vi "Three Motor Mover.vi"() -> ()   [LabVIEW 2019]
panel:
  in  "Low 1":dbl=-100.0 format="%.1f"
  in  "High 1":dbl=100.0 format="%.1f"
  in  "Low 2":dbl=-100.0 format="%.1f"
  in  "High 2":dbl=100.0 format="%.1f"
  in  "Low 3":dbl=-100.0 format="%.1f"
  in  "High 3":dbl=100.0 format="%.1f"
  in  "Zero 3":bool
  in  "Zero 2":bool
  in  "Zero 1":bool
  out "Position 3":dbl format="%.4f"
  in  "Backward Big 3":bool
  in  "Forward Big 3":bool
  in  "Backward Small 3":bool
  in  "Forward Small 3":bool
  in  "Motor 3":refnum<visa-resource-name>="ASRL6::INSTR"
  in  "Large Step Size 3":dbl=10.0 format="%.1f"
  in  "Small Step Size 3":dbl=1.0 format="%_2f"
  out "Position 2":dbl format="%.4f"
  in  "Backward Big 2":bool
  in  "Forward Big 2":bool
  in  "Backward Small 2":bool
  in  "Forward Small 2":bool
  in  "Motor 2":refnum<visa-resource-name>="ASRL5::INSTR"
  in  "Large Step Size 2":dbl=10.0 format="%.1f"
  in  "Small Step Size 2":dbl=1.0 format="%_2f"
  out "Position 1":dbl format="%.4f"
  in  "stop":bool
  in  "Backward Big 1":bool
  in  "Forward Big 1":bool
  in  "Backward Small 1":bool
  in  "Forward Small 1":bool
  in  "Motor 1":refnum<visa-resource-name>="ASRL4::INSTR"
  in  "Large Step Size 1":dbl=10.0 format="%.1f"
  in  "Small Step Size 1":dbl=1.0 format="%_2f"
  # "Limits"
  # "Limits"
  # "Limits"
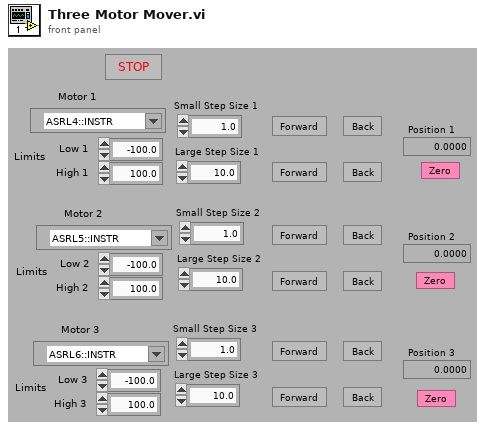
[diagram p1: front panel]
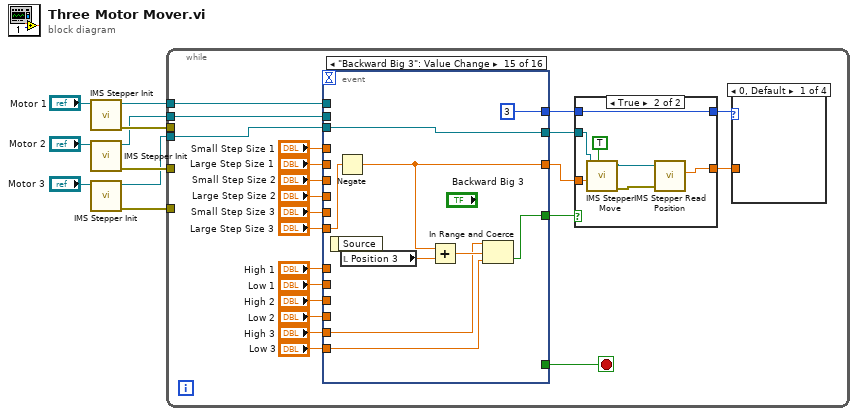
[diagram p0: block diagram]
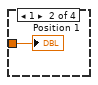
[diagram p2: hidden frame]
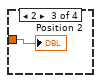
[diagram p3: hidden frame]
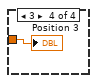
[diagram p4: hidden frame]
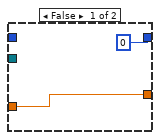
[diagram p5: hidden frame]
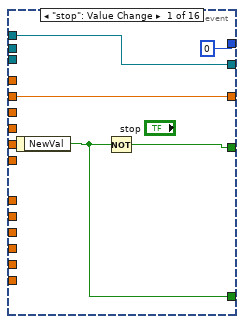
[diagram p6: hidden frame]
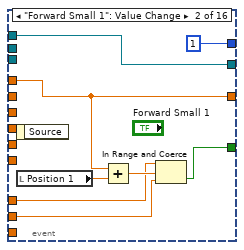
[diagram p7: hidden frame]
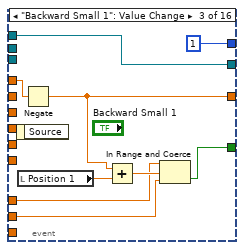
[diagram p8: hidden frame]
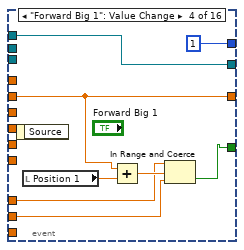
[diagram p9: hidden frame]
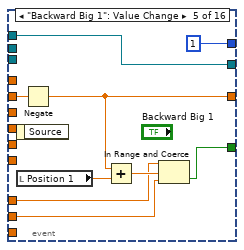
[diagram p10: hidden frame]
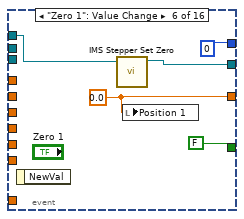
[diagram p11: hidden frame]
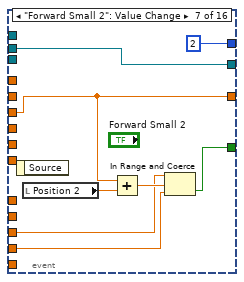
[diagram p12: hidden frame]
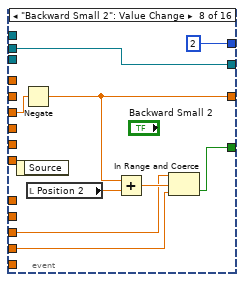
[diagram p13: hidden frame]
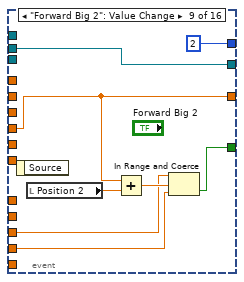
[diagram p14: hidden frame]
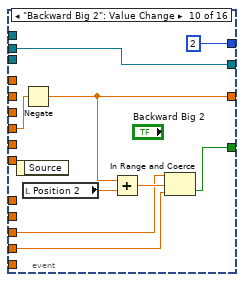
[diagram p15: hidden frame]
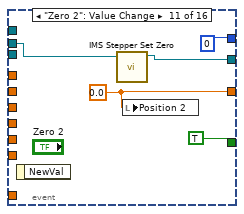
[diagram p16: hidden frame]
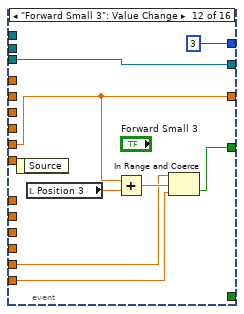
[diagram p17: hidden frame]
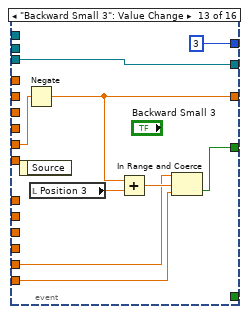
[diagram p18: hidden frame]
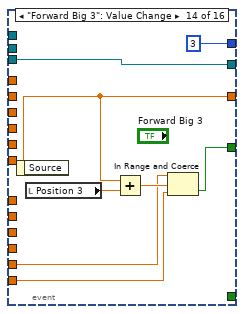
[diagram p19: hidden frame]
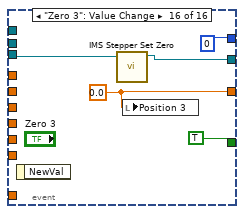
[diagram p20: hidden frame]
diagram:
  n1 = call "IMS Stepper Init.vi"("Instrument Address"="Motor 1") -> ("error out"=w9:errorcluster, "dup VISA Resource Name"=w5:refnum<visa-resource-name>)  [unwired: 4 in, 1 out]
  n2 = call "IMS Stepper Init.vi"("Instrument Address"="Motor 2") -> ("error out"=w7:errorcluster, "dup VISA Resource Name"=w3:refnum<visa-resource-name>)  [unwired: 4 in, 1 out]
  n3 = call "IMS Stepper Init.vi"("Instrument Address"="Motor 3") -> ("error out"=w8:errorcluster, "dup VISA Resource Name"=w1:refnum<visa-resource-name>)  [unwired: 4 in, 1 out]
  n4 = while {
    tunnel: w5 -> [w24]
    tunnel: w9 -> [_]
    tunnel: w8 -> [_]
    tunnel: w7 -> [_]
    tunnel: w3 -> [w22]
    tunnel: w1 -> [w21]
    stop <- w16 stop-if-true
    n5 = event shown="[14] \"Backward Big 3\": Value Change" {
      selector: _ -> [_ _ _ _ _ _ _ _ _ _ _ _ _ _ _ _]
      dyn-events: _ -> [_ _ _ _ _ _ _ _ _ _ _ _ _ _ _ _]
      timeout: _ -> [_ _ _ _ _ _ _ _ _ _ _ _ _ _ _ _]
      tunnel: w24 -> [w47 w56 w65 w73 w81 w84 _ _ _ _ _ _ _ _ _ _]
      tunnel: "Small Step Size 1" -> [_ w53 w63 _ _ _ _ _ _ _ _ _ _ _ _ _]
      tunnel: "Large Step Size 1" -> [w46 _ _ w66 w82 _ _ _ _ _ _ _ _ _ _ _]
      tunnel: [w47 w56 w65 w73 w81 w83 w94 w103 w111 w119 w122 w133 w141 w150 w158 w161] -> w31
      tunnel: [w46 w53 w59 w66 w76 w85 w90 w98 w107 w115 w124 w130 w138 w147 w154 w163] -> w30
      tunnel: [w45 w49 w60 w67 w77 FALSE ("NewVal") w91 w99 w108 w116 TRUE ("NewVal") w127 w135 w146 w155 TRUE ("NewVal")] -> w23
      tunnel: [0 1 1 1 1 0 2 2 2 2 0 3 3 3 3 0] -> w27
      tunnel: w22 -> [_ _ _ _ _ _ w94 w103 w111 w119 w123 _ _ _ _ _]
      tunnel: w21 -> [_ _ _ _ _ _ _ _ _ _ _ w133 w141 w150 w158 w162]
      tunnel: "Small Step Size 2" -> [_ _ _ _ _ _ w90 w102 _ _ _ _ _ _ _ _]
      tunnel: "Large Step Size 2" -> [_ _ _ _ _ _ _ _ w107 w120 _ _ _ _ _ _]
      tunnel: "Small Step Size 3" -> [_ _ _ _ _ _ _ _ _ _ _ w130 w142 _ _ _]
      tunnel: "Large Step Size 3" -> [_ _ _ _ _ _ _ _ _ _ _ _ _ w147 w159 _]
      tunnel: "High 1" -> [_ w51 w58 w69 w75 _ _ _ _ _ _ _ _ _ _ _]
      tunnel: "Low 1" -> [_ w50 w57 w68 w74 _ _ _ _ _ _ _ _ _ _ _]
      tunnel: "High 2" -> [_ _ _ _ _ _ w89 w97 w106 w114 _ _ _ _ _ _]
      tunnel: "Low 2" -> [_ _ _ _ _ _ w88 w96 w105 w113 _ _ _ _ _ _]
      tunnel: "High 3" -> [_ _ _ _ _ _ _ _ _ _ _ w129 w137 w145 w153 _]
      tunnel: "Low 3" -> [_ _ _ _ _ _ _ _ _ _ _ w128 w136 w144 w152 _]
      tunnel: [w44 _ _ _ _ _ _ _ _ _ _ _ _ _ _ _] -> w16
      event "stop": Value Change {
        n6 = event-data() -> ("NewVal"=w44:bool)  [unwired: 1 in]
        n7 = Not(x=w44) -> (.not. x?=w45:bool)
      }
      event "Forward Small 1": Value Change {
        n8 = event-data() -> ()  [unwired: 1 in, 1 out]
        n9 = local read "Position 1"() -> (w54:dbl)
        n10 = Add(x=w53, y=w54) -> (x+y=w52:dbl)
        n11 = In Range and Coerce(upper limit=w51, x=w52, lower limit=w50) -> (In Range?=w49:bool)  [unwired: 1 out]
      }
      event "Backward Small 1": Value Change {
        n12 = event-data() -> ()  [unwired: 1 in, 1 out]
        n13 = local read "Position 1"() -> (w61:dbl)
        n14 = Negate(x=w63) -> (-x=w59:dbl)
        n15 = Add(x=w59, y=w61) -> (x+y=w62:dbl)
        n16 = In Range and Coerce(upper limit=w58, x=w62, lower limit=w57) -> (In Range?=w60:bool)  [unwired: 1 out]
      }
      event "Forward Big 1": Value Change {
        n17 = event-data() -> ()  [unwired: 1 in, 1 out]
        n18 = local read "Position 1"() -> (w70:dbl)
        n19 = Add(x=w66, y=w70) -> (x+y=w71:dbl)
        n20 = In Range and Coerce(upper limit=w69, x=w71, lower limit=w68) -> (In Range?=w67:bool)  [unwired: 1 out]
      }
      event "Backward Big 1": Value Change {
        n21 = event-data() -> ()  [unwired: 1 in, 1 out]
        n22 = local read "Position 1"() -> (w78:dbl)
        n23 = Negate(x=w82) -> (-x=w76:dbl)
        n24 = Add(x=w76, y=w78) -> (x+y=w79:dbl)
        n25 = In Range and Coerce(upper limit=w75, x=w79, lower limit=w74) -> (In Range?=w77:bool)  [unwired: 1 out]
      }
      event "Zero 1": Value Change {
        w85 = 0.0 ("Large Step Size 3")
        n26 = event-data() -> ()  [unwired: 1 in, 1 out]
        n27 = call "IMS Stepper Set Zero.vi"("Instrument Address"=w84) -> ("Instrument Address Out"=w83:refnum<visa-resource-name>)  [unwired: 4 in, 1 out]
        n28 = local write "Position 1"(w85) -> ()
      }
      event "Forward Small 2": Value Change {
        n29 = event-data() -> ()  [unwired: 1 in, 1 out]
        n30 = local read "Position 2"() -> (w92:dbl)
        n31 = Add(x=w90, y=w92) -> (x+y=w93:dbl)
        n32 = In Range and Coerce(upper limit=w89, x=w93, lower limit=w88) -> (In Range?=w91:bool)  [unwired: 1 out]
      }
      event "Backward Small 2": Value Change {
        n33 = event-data() -> ()  [unwired: 1 in, 1 out]
        n34 = Negate(x=w102) -> (-x=w98:dbl)
        n35 = local read "Position 2"() -> (w100:dbl)
        n36 = Add(x=w98, y=w100) -> (x+y=w101:dbl)
        n37 = In Range and Coerce(upper limit=w97, x=w101, lower limit=w96) -> (In Range?=w99:bool)  [unwired: 1 out]
      }
      event "Forward Big 2": Value Change {
        n38 = event-data() -> ()  [unwired: 1 in, 1 out]
        n39 = local read "Position 2"() -> (w109:dbl)
        n40 = Add(x=w107, y=w109) -> (x+y=w110:dbl)
        n41 = In Range and Coerce(upper limit=w106, x=w110, lower limit=w105) -> (In Range?=w108:bool)  [unwired: 1 out]
      }
      event "Backward Big 2": Value Change {
        n42 = event-data() -> ()  [unwired: 1 in, 1 out]
        n43 = Negate(x=w120) -> (-x=w115:dbl)
        n44 = local read "Position 2"() -> (w117:dbl)
        n45 = Add(x=w115, y=w117) -> (x+y=w118:dbl)
        n46 = In Range and Coerce(upper limit=w114, x=w118, lower limit=w113) -> (In Range?=w116:bool)  [unwired: 1 out]
      }
      event "Zero 2": Value Change {
        w124 = 0.0 ("Large Step Size 3")
        n47 = event-data() -> ()  [unwired: 1 in, 1 out]
        n48 = call "IMS Stepper Set Zero.vi"("Instrument Address"=w123) -> ("Instrument Address Out"=w122:refnum<visa-resource-name>)  [unwired: 4 in, 1 out]
        n49 = local write "Position 2"(w124) -> ()
      }
      event "Forward Small 3": Value Change {
        n50 = event-data() -> ()  [unwired: 1 in, 1 out]
        n51 = local read "Position 3"() -> (w131:dbl)
        n52 = Add(x=w130, y=w131) -> (x+y=w132:dbl)
        n53 = In Range and Coerce(upper limit=w129, x=w132, lower limit=w128) -> (In Range?=w127:bool)  [unwired: 1 out]
      }
      event "Backward Small 3": Value Change {
        n54 = event-data() -> ()  [unwired: 1 in, 1 out]
        n55 = Negate(x=w142) -> (-x=w138:dbl)
        n56 = local read "Position 3"() -> (w139:dbl)
        n57 = Add(x=w138, y=w139) -> (x+y=w140:dbl)
        n58 = In Range and Coerce(upper limit=w137, x=w140, lower limit=w136) -> (In Range?=w135:bool)  [unwired: 1 out]
      }
      event "Forward Big 3": Value Change {
        n59 = event-data() -> ()  [unwired: 1 in, 1 out]
        n60 = local read "Position 3"() -> (w148:dbl)
        n61 = Add(x=w147, y=w148) -> (x+y=w149:dbl)
        n62 = In Range and Coerce(upper limit=w145, x=w149, lower limit=w144) -> (In Range?=w146:bool)  [unwired: 1 out]
      }
      event "Backward Big 3": Value Change {
        n63 = event-data() -> ()  [unwired: 1 in, 1 out]
        n64 = Negate(x=w159) -> (-x=w154:dbl)
        n65 = local read "Position 3"() -> (w156:dbl)
        n66 = Add(x=w154, y=w156) -> (x+y=w157:dbl)
        n67 = In Range and Coerce(upper limit=w153, x=w157, lower limit=w152) -> (In Range?=w155:bool)  [unwired: 1 out]
      }
      event "Zero 3": Value Change {
        w163 = 0.0 ("Large Step Size 3")
        n68 = event-data() -> ()  [unwired: 1 in, 1 out]
        n69 = call "IMS Stepper Set Zero.vi"("Instrument Address"=w162) -> ("Instrument Address Out"=w161:refnum<visa-resource-name>)  [unwired: 4 in, 1 out]
        n70 = local write "Position 3"(w163) -> ()
      }
    }
    n71 = case shown="True" w23 {
      tunnel: w31 -> [_ w38]
      tunnel: w30 -> [w35 w41]
      tunnel: [w35 w40] -> w25
      tunnel: [0 w39] -> w26
      tunnel: w27 -> [_ w39]
      frame False {
      }
      frame True {
        n72 = call "IMS Stepper Move.vi"("Mode"=TRUE, "Distance"=w41, "Instrument Address"=w38) -> ("error out"=w43:errorcluster, "Instrument Address Out"=w37:refnum<visa-resource-name>)  [unwired: 4 in]
        n73 = call "IMS Stepper Read Position.vi"("Instrument Address"=w37, "error in (no error)"=w43) -> ("Response"=w40:dbl)  [unwired: 2 in, 2 out]
      }
    }
    n74 = case shown="0, Default" w26 {
      tunnel: w25 -> [_ w32 w33 w34]
      frame 0, Default {
      }
      frame 1 {
        "Position 1" <- w32
      }
      frame 2 {
        "Position 2" <- w33
      }
      frame 3 {
        "Position 3" <- w34
      }
    }
  }
